vi "RM.deleteDeviceReservationDB.vi"(8 "error in":errorcluster, 10 "device name":string="deviceName", 11 "Item Ref in":T1 format="%.0x") -> (0 "error out":errorcluster, 1 "found":bool, 3 "Item Ref out":T1 format="%.0x")   [LabVIEW 2016, in "FPGA Addon Shared.lvlib"]
uses:
  FPGA Addon Shared.lvlib
  <vilib>/NI Veristand/Custom Device API/Custom Device Item Ref.ctl
  <vilib>/NI Veristand/Custom Device API/Get Item Property (Variant).vi
  <vilib>/NI Veristand/Custom Device API/Set Item Property (Variant).vi
  <vilib>/NI VeriStand/Custom Device Tools/Custom Device Utility Library/Custom Device Utility Library.lvlib
  <vilib>/NI VeriStand/Custom Device API/Custom Device API.lvlib
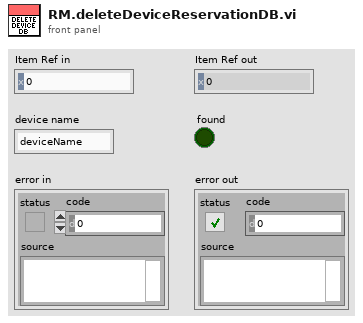
[diagram p1: front panel]
types:
  T1 = typedef "Custom Device API.lvlib/Custom Device Item Ref.ctl" = u64
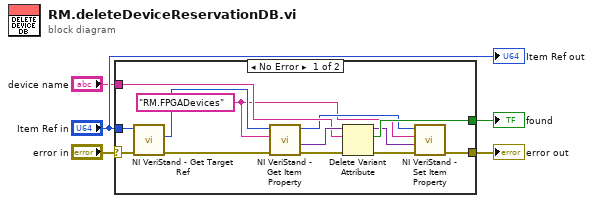
[diagram p0: block diagram]
diagram:
  n1 = case shown="No Error" "error in" {
    selector: "error in" -> [w14 w19]
    tunnel: "Item Ref in" -> [w18 _]
    tunnel: [w15 _] -> w1
    tunnel: [w7 w19] -> w4
    tunnel: "device name" -> [w11 _]
    frame No Error {
      w9 = "RM.FPGADevices" ("Property Name")
      n2 = call <vilib>:"NI VeriStand - Get Target Ref.vi"("error in"=w14, "Item Ref in"=w18) -> ("error out"=w13:errorcluster, "Target Ref"=w17:T1)  [unwired: 6 in, 2 out]
      n3 = call-poly <vilib>:"NI VeriStand - Get Item Property.vi"("error in (no error)"=w13, "Property Name"=w9, "Item Ref in"=w17) -> ("error out"=w12:errorcluster, "Value"=w16:variant, "Item Ref out"=w10:T1)  [unwired: 5 in, 1 out]
      n4 = Delete Variant Attribute(4:w12, 6:w11, 7:w16) -> (0:w8:errorcluster, 2:w15:bool, 3:w6:variant)
      n5 = call-poly <vilib>:"NI VeriStand - Set Item Property.vi"("error in (no error)"=w8, "Value"=w6, "Property Name"=w9, "Item Ref in"=w10) -> ("error out"=w7:errorcluster)  [unwired: 5 in, 2 out]
    }
    frame Error {
    }
  }
  "found" <- w1
  "error out" <- w4
  "Item Ref out" <- "Item Ref in"
